vi "Word_Clear_Document.vi"(0 "Word._Document":refnum<k7>, 11 "error in":errorcluster) -> (15 "error out":errorcluster)   [LabVIEW 2017, in "NI_ReportGenerationToolkit.lvlib"]
uses:
  <vilib>/addons/_office/NI_ReportGenerationToolkit.lvlib
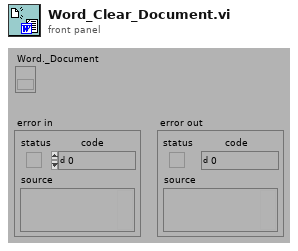
[diagram p1: front panel]
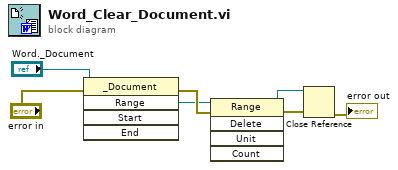
[diagram p0: block diagram]
diagram:
  n1 = invoke class="_Document" method="Range"(reference="Word._Document", error in="error in") -> (error out=w3:errorcluster, "Range"=w2:refnum<k7>)  [unwired: 3 in, 3 out]
  n2 = invoke class="Range" method="Delete"(reference=w2, error in=w3) -> (reference out=w5:refnum<k7>, error out=w4:errorcluster)  [unwired: 3 in, 3 out]
  n3 = Close Reference(reference=w5, error in (no error)=w4) -> (error out=→"error out":errorcluster)
